vi "Measure Q.vi"(8 "error in (no error)":errorcluster, 11 "Hardware Parameters":T1={"Scan Calibration [G/V]"=0.0, "Modulation Calibration [G/V]"=0.0, "Modulation Phase [deg]"=0.0, "Modulation Frequency [Hz]"=0.0, "Attenuation [dB]"=0, "Input Channel Count"=0, "Time constant"=7, "Sensitivity"=17, "Frequency Output Voltage [V]"=0.0, "Phase Output Voltage [V]"=0.0, "Lock-in Offset Compensation"=FALSE, "RF [GHz]"=0.0, "Q Start"=0.0, "Q End"=0.0, "Balance"=0.0, "Phase Error"=0.0, "AFC Error"=0.0, "AFC"=FALSE, "Magnet Rotation"=FALSE, "Balance Scaling Factor"=1.0, "Phase Error Scaling Factor"=1.0, "AFC Error Scaling Factor"=1.0, "Frequency Counter ID"="", "Sweep Waveform"=enum."Sawtooth", "Q-Factor Scale"=0.0, " Q-Data Scale"=0.0, " Q-Data Offset"=0.0, "Magnet Rotation Slope"=0.0, "Magnet Rotation Offset"=0.0, "Phase Sweep Resolution"=0.0, "Hardware Version Number"="", "Spectrometer ID Number"=0, "Spectrometer Name"="", "Lock in Saturation"=0.0, "Balance Threshold"=0.0, "Phase Error Threshold"=0.0, "AFC Error Threshold"=0.0, "Linear Actuator Length"=0.0, "Lock-in OK?"=FALSE, "Ignore Lock-in Comm. Failure"=FALSE, "Gradient Addresses"=[], "Gradient Calibrations [G/A*mm]"=[], "Gradient Power Supplies"=[], "Lock-in Address"="", "Magnet Type"=enum."RRI", "Camera Names"=[], "Sweep Limit [Gauss]"=0.0, "Modulation Limit [Gauss]"=0.0, "Balance Threshold Exceeded?"=FALSE, "Phase Threshold Exceeded?"=FALSE, "AFC Threshold Exceeded?"=FALSE, "Consecutive Re-tune attempts"=0, "Reverse Sweep Slope [sec]"=0.0, "Reverse Sweep Offset [G]"=0.0, "AFC Field Correction [V/MHz]"=0.0, "Active Gradients (X Y Z)"=[], "SpO2 Calibration [SpO2/V]"=1.0, "Heart Rate Calibration [BPM/V]"=1.0, "Thermocouple Channel"=""} {"Sensitivity" items=["", "2 nV", "5 nV", "10 nV", "20 nV", "50 nV", "100 nV", "200 nV", "500 nV", "1 uV", "2 uV", "5 uV", "10 uV", "20 uV", "50 uV", "100 uV", "200 uV", "500 uV", "1 mV", "2 mV", "5 mV", "10 mV", "20 mV", "50 mV", "100 mV", "200 mV", "500 mV", "1 V"]; "Time constant" items=["10 us", "20 us", "40 us", "80 us", "160 us", "320 us", "640 us", "5 ms", "10 ms", "20 ms", "50 ms", "100 ms", "200 ms", "500 ms", "1 s", "2 s", "5 s", "10 s", "20 s", "50 s", "100 s", "200 s", "500 s", "1 ks", "2 ks", "5 ks", "10 ks", "20 ks", "50 ks", "100 ks"]}) -> (0 "error out":errorcluster, 2 "Q Factor":dbl, 3 "Hardware Parameters Out":T1={"Scan Calibration [G/V]"=0.0, "Modulation Calibration [G/V]"=0.0, "Modulation Phase [deg]"=0.0, "Modulation Frequency [Hz]"=0.0, "Attenuation [dB]"=0, "Input Channel Count"=0, "Time constant"=7, "Sensitivity"=17, "Frequency Output Voltage [V]"=0.0, "Phase Output Voltage [V]"=0.0, "Lock-in Offset Compensation"=FALSE, "RF [GHz]"=0.0, "Q Start"=0.0, "Q End"=0.0, "Balance"=0.0, "Phase Error"=0.0, "AFC Error"=0.0, "AFC"=FALSE, "Magnet Rotation"=FALSE, "Balance Scaling Factor"=1.0, "Phase Error Scaling Factor"=1.0, "AFC Error Scaling Factor"=1.0, "Frequency Counter ID"="", "Sweep Waveform"=enum."Sawtooth", "Q-Factor Scale"=0.0, " Q-Data Scale"=0.0, " Q-Data Offset"=0.0, "Magnet Rotation Slope"=0.0, "Magnet Rotation Offset"=0.0, "Phase Sweep Resolution"=0.0, "Hardware Version Number"="", "Spectrometer ID Number"=0, "Spectrometer Name"="", "Lock in Saturation"=0.0, "Balance Threshold"=0.0, "Phase Error Threshold"=0.0, "AFC Error Threshold"=0.0, "Linear Actuator Length"=0.0, "Lock-in OK?"=FALSE, "Ignore Lock-in Comm. Failure"=FALSE, "Gradient Addresses"=[], "Gradient Calibrations [G/A*mm]"=[], "Gradient Power Supplies"=[], "Lock-in Address"="", "Magnet Type"=enum."RRI", "Camera Names"=[], "Sweep Limit [Gauss]"=0.0, "Modulation Limit [Gauss]"=0.0, "Balance Threshold Exceeded?"=FALSE, "Phase Threshold Exceeded?"=FALSE, "AFC Threshold Exceeded?"=FALSE, "Consecutive Re-tune attempts"=0, "Reverse Sweep Slope [sec]"=0.0, "Reverse Sweep Offset [G]"=0.0, "AFC Field Correction [V/MHz]"=0.0, "Active Gradients (X Y Z)"=[], "SpO2 Calibration [SpO2/V]"=1.0, "Heart Rate Calibration [BPM/V]"=1.0, "Thermocouple Channel"=""} {"Sensitivity" items=["", "2 nV", "5 nV", "10 nV", "20 nV", "50 nV", "100 nV", "200 nV", "500 nV", "1 uV", "2 uV", "5 uV", "10 uV", "20 uV", "50 uV", "100 uV", "200 uV", "500 uV", "1 mV", "2 mV", "5 mV", "10 mV", "20 mV", "50 mV", "100 mV", "200 mV", "500 mV", "1 V"]; "Time constant" items=["10 us", "20 us", "40 us", "80 us", "160 us", "320 us", "640 us", "5 ms", "10 ms", "20 ms", "50 ms", "100 ms", "200 ms", "500 ms", "1 s", "2 s", "5 s", "10 s", "20 s", "50 s", "100 s", "200 s", "500 s", "1 ks", "2 ks", "5 ks", "10 ks", "20 ks", "50 ks", "100 ks"]})   [LabVIEW 2016]
uses:
  Types/Hardware Parameters.ctl
  <vilib>/Analysis/baseanly.llb/Mean (DBL).vi
  <vilib>/Analysis/NI_AALBase.lvlib
panel:
  out "size(s)":i32
  out "Frequency Voltage":dbl
  in  "Narrow sweep":dbl=1.0
  out "Voltage Input":dbl=9.98
  in  "Wide sweep":dbl=10.0
  out "XY Graph":cluster{"Y":dbl[], "Y":dbl[]}[](graph)
  out "Balance":dbl=-3.95030517578125
  # "Bridge I/O"
  # "Magnet Rotation"
  # "Field Calibration"
  # "Lock In Amplifier"
  # "Spectrometer Information"
  # "DAQ Settings"
  # "Gradient Coils and Field"
  # "X"
  # "Y"
  # "Z"
  # "Q-Measurements"
  # "Bridge I/O"
  # "Magnet Rotation"
  # "Field Calibration"
  # "Lock In Amplifier"
  # "Spectrometer Information"
  # "DAQ Settings"
  # "Gradient Coils and Field"
  # "X"
  # "Y"
  # "Z"
  # "Q-Measurements"
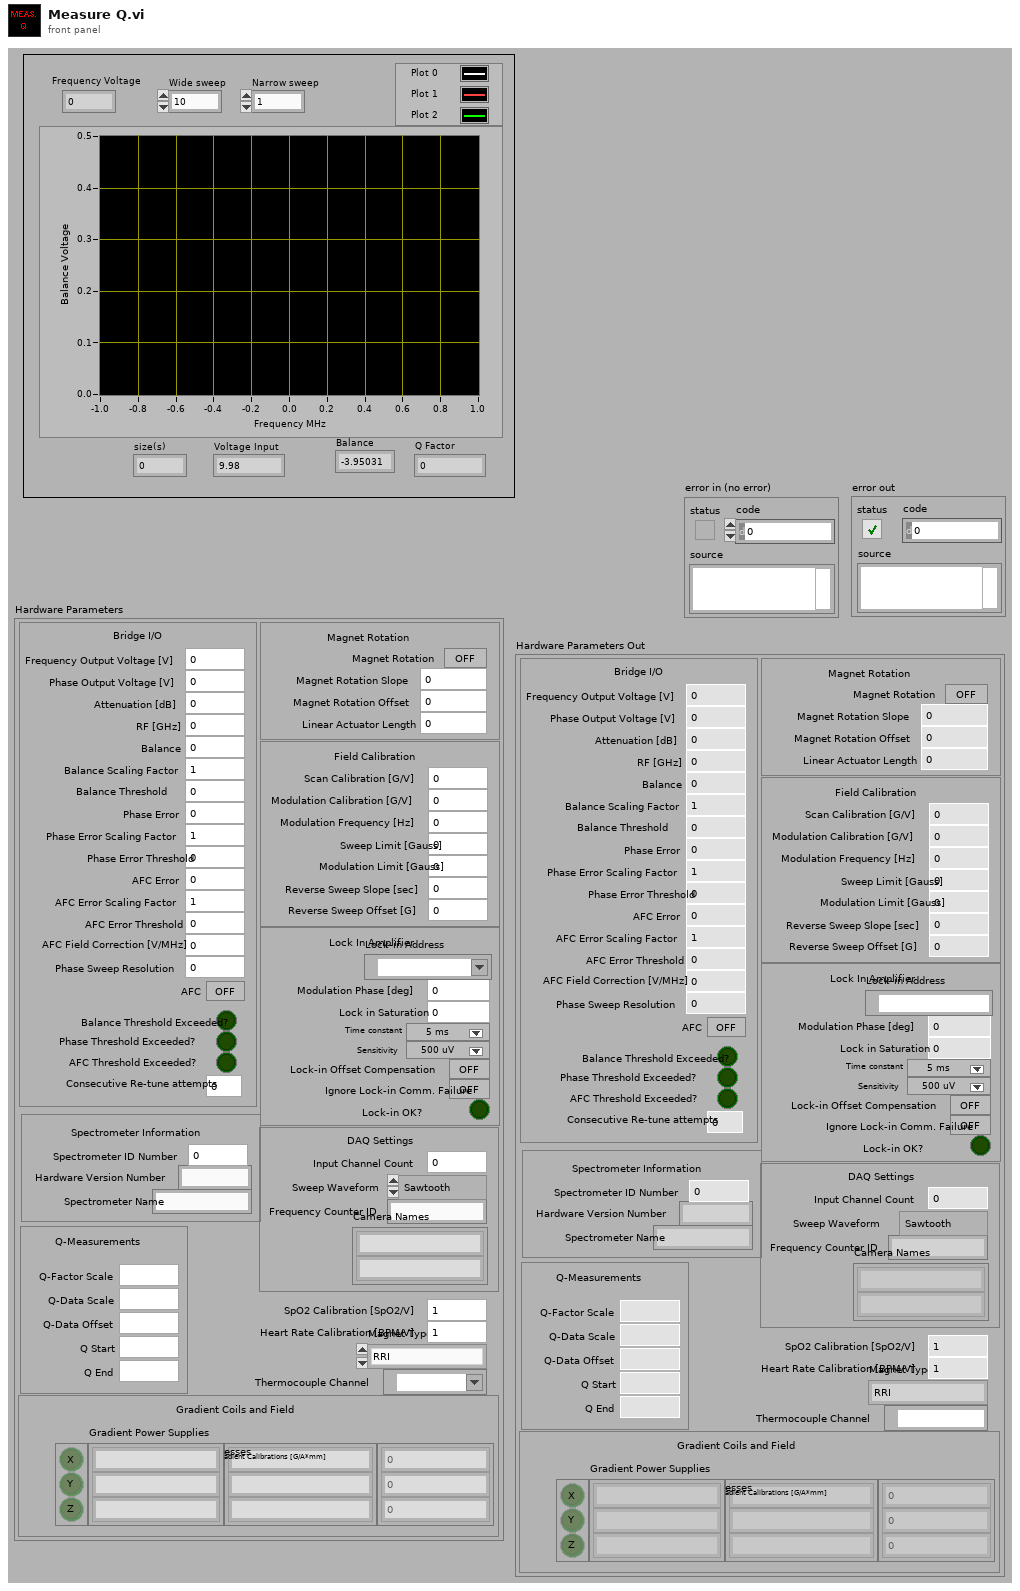
[diagram p1: front panel]
types:
  T1 = typedef "Hardware Parameters.ctl" = cluster{"Scan Calibration [G/V]":dbl, "Modulation Calibration [G/V]":dbl, "Modulation Phase [deg]":dbl, "Modulation Frequency [Hz]":dbl, "Attenuation [dB]":u16, "Input Channel Count":i32, "Time constant":u16, "Sensitivity":u16, "Frequency Output Voltage [V]":dbl, "Phase Output Voltage [V]":dbl, "Lock-in Offset Compensation":bool, "RF [GHz]":dbl, "Q Start":dbl, "Q End":dbl, "Balance":dbl, "Phase Error":dbl, "AFC Error":dbl, "AFC":bool, "Magnet Rotation":bool, "Balance Scaling Factor":dbl, "Phase Error Scaling Factor":dbl, "AFC Error Scaling Factor":dbl, "Frequency Counter ID":string, "Sweep Waveform":enum16{"Sine Wave", "Square Wave", "Sawtooth", "Triangle Wave"}, "Q-Factor Scale":dbl, " Q-Data Scale":dbl, " Q-Data Offset":dbl, "Magnet Rotation Slope":dbl, "Magnet Rotation Offset":dbl, "Phase Sweep Resolution":dbl, "Hardware Version Number":string, "Spectrometer ID Number":i32, "Spectrometer Name":string, "Lock in Saturation":dbl, "Balance Threshold":dbl, "Phase Error Threshold":dbl, "AFC Error Threshold":dbl, "Linear Actuator Length":dbl, "Lock-in OK?":bool, "Ignore Lock-in Comm. Failure":bool, "Gradient Addresses":string[], "Gradient Calibrations [G/A*mm]":dbl[], "Gradient Power Supplies":string[], "Lock-in Address":refnum<visa-resource-name>, "Magnet Type":enum16{"RRI", "BARDA", "Whole Body Permanent", "RRI Electromagnet"}, "Camera Names":string[], "Sweep Limit [Gauss]":dbl, "Modulation Limit [Gauss]":dbl, "Balance Threshold Exceeded?":bool, "Phase Threshold Exceeded?":bool, "AFC Threshold Exceeded?":bool, "Consecutive Re-tune attempts":i32, "Reverse Sweep Slope [sec]":dbl, "Reverse Sweep Offset [G]":dbl, "AFC Field Correction [V/MHz]":dbl, "Active Gradients (X Y Z)":bool[], "SpO2 Calibration [SpO2/V]":dbl, "Heart Rate Calibration [BPM/V]":dbl, "Thermocouple Channel":tag}
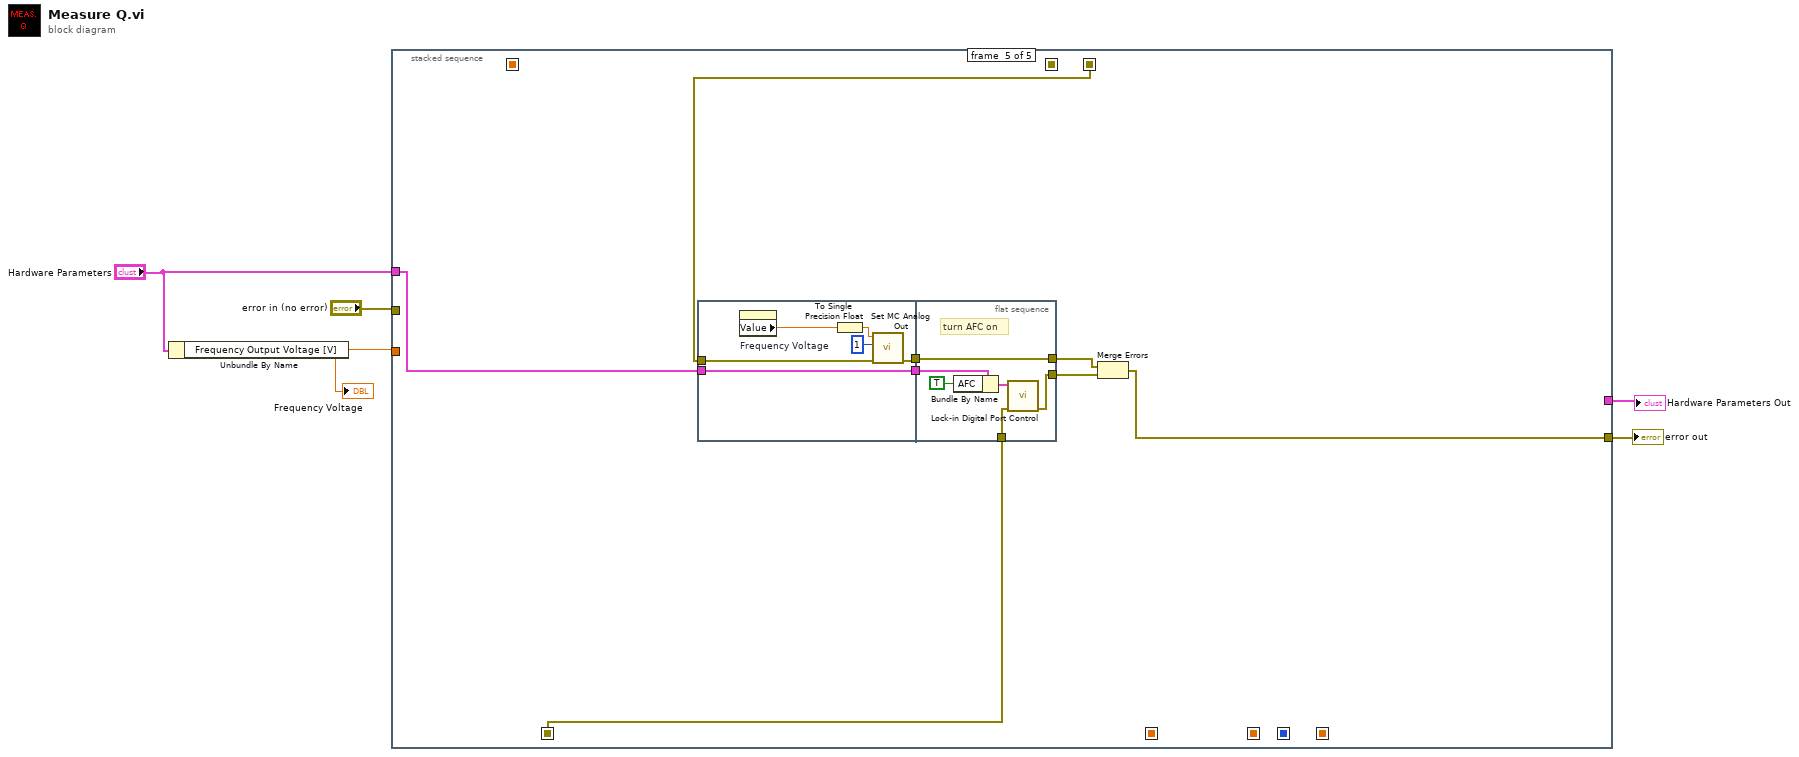
[diagram p0: block diagram]
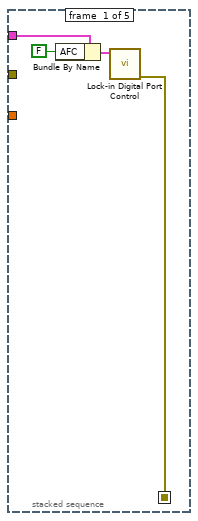
[diagram p2: hidden frame]
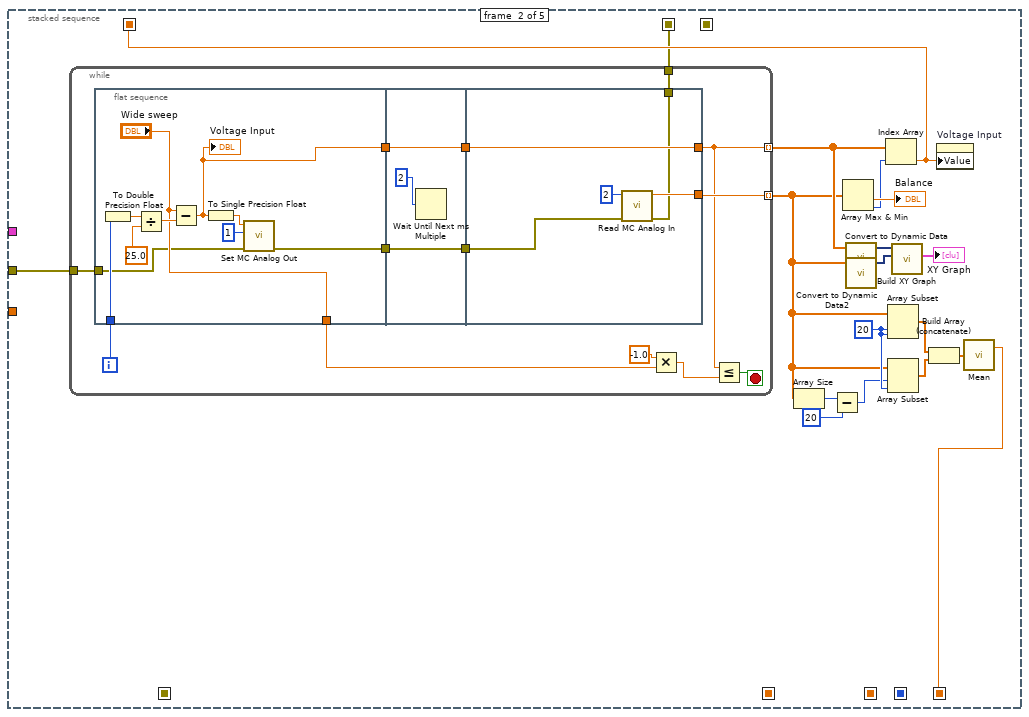
[diagram p3: hidden frame]
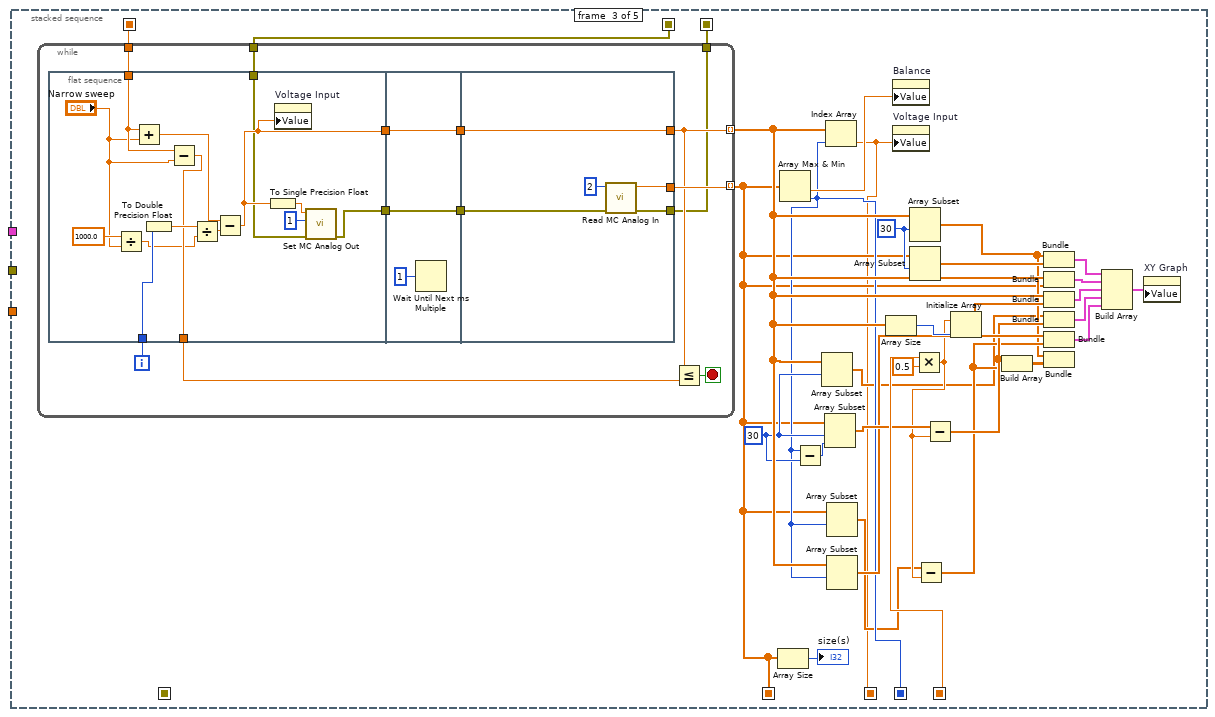
[diagram p4: hidden frame]
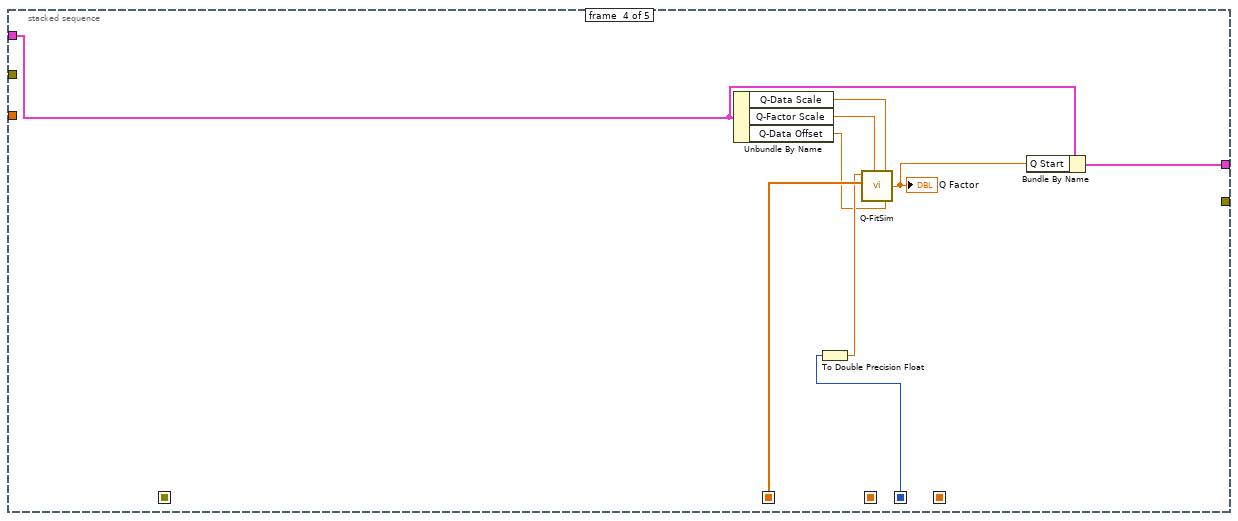
[diagram p5: hidden frame]
diagram:
  n1 = Unbundle By Name("Hardware Parameters") -> ("Frequency Output Voltage [V]"=w4:dbl)
  "Frequency Voltage" <- w4
  n2 = stacked-sequence {
    seq-local: [_ _ w61 _ _] -> [_ _ _ _ _]
    seq-local: [_ w16 _ _ _] -> [_ _ w79 _ _]
    seq-local: [_ w17 _ _ _] -> [_ _ w84 _ _]
    seq-local: [_ _ w62 _ _] -> [_ _ _ w133 _]
    seq-local: [_ _ w65 _ _] -> [_ _ _ w132 _]
    seq-local: [_ w10 _ _ _] -> [_ _ w60 _ _]
    seq-local: [_ _ w59 _ _] -> [_ _ _ _ w141]
    seq-local: [w6 _ _ _ _] -> [_ _ _ _ w138]
    tunnel: w4 -> [_ _ _ _ _]
    tunnel: "error in (no error)" -> [_ w11 _ _ _]
    tunnel: "Hardware Parameters" -> [w9 _ _ w127 w139]
    tunnel: [_ _ _ w125 _] -> w2
    tunnel: [_ _ _ _ w134] -> w1
    frame #0 {
      n3 = Bundle By Name(cluster=w9, "AFC"=FALSE) -> (w8:T1)
      n4 = call "Lock-in Digital Port Control.vi"("Hardware Parameters"=w8) -> ("error out"=w6:errorcluster)  [unwired: 10 in]
    }
    frame #1 {
      w20 = 20 ("index")
      n5 = while {
        tunnel: [w39] -> w12 mode=indexing
        tunnel: [w35] -> w18 mode=indexing
        tunnel: w11 -> [w31]
        tunnel: [w28] -> w10
        i -> [w40]
        stop <- w34 stop-if-true
        n6 = flat-sequence {
          tunnel: [w43] -> w33
          tunnel: ["Wide sweep"] -> w38
          tunnel: w40 -> [w50]
          tunnel: w31 -> [w42]
          tunnel: [w41] -> w29
          tunnel: w33 -> [w53]
          tunnel: [w53] -> w32
          tunnel: [w51] -> w30
          tunnel: w29 -> [w51]
          tunnel: [w56] -> w39
          tunnel: w32 -> [w58]
          tunnel: [w58] -> w35
          tunnel: w30 -> [w55]
          tunnel: [w54] -> w28
          frame #0 {
            n7 = To Double Precision Float(number=w50) -> (double precision float=w47:dbl)
            n8 = Divide(x=w47, y=25.0) -> (x/y=w49:dbl)
            n9 = Subtract(x="Wide sweep", y=w49) -> (x-y=w43:dbl)
            "Voltage Input" <- w43
            n10 = To Single Precision Float(number=w43) -> (single precision float=w44:sgl)
            n11 = call "Set MC Analog Out.vi"("error in (no error)"=w42, "Channel"=1, "Output Voltage"=w44) -> ("error out"=w41:errorcluster)  [unwired: 8 in]
          }
          frame #1 {
            n12 = Wait Until Next ms Multiple(millisecond multiple=u32 2 ("Inner Loop")) -> ()  [unwired: 1 out]
          }
          frame #2 {
            n13 = call "Read MC Analog In.vi"("error in (no error)"=w55, "channel"=2) -> ("error out"=w54:errorcluster, "Voltage Input"=w56:dbl)  [unwired: 8 in]
          }
        }
        n14 = Multiply(x=-1.0, y=w38) -> (x*y=w37:dbl)
        n15 = Less Or Equal?(x=w35, y=w37) -> (x <= y?=w34:bool)
      }
      n16 = Array Size(array=w12) -> (size(s)=w15:i32)
      n17 = Subtract(x=w15, y=20) -> (x-y=w13:i32)
      n18 = Array Max & Min(array=w12) -> (min value=→"Balance":dbl, min index (indices)=w23:i32)  [unwired: 2 out]
      n19 = call "Convert to Dynamic Data"("Array"=w18) -> ("Dynamic Data Type"=w25:dynamicdata)  [unwired: 3 out]
      n20 = call "Convert to Dynamic Data2"("Array"=w12) -> ("Dynamic Data Type"=w26:dynamicdata)  [unwired: 3 out]
      n21 = Index Array(array=w18, index=w23) -> (element=w17:dbl)
      n22 = Array Subset(array=w12, index=w20, length=w20) -> (w21:dbl[])
      n23 = Array Subset(array=w12, index=w13, length=w20) -> (w22:dbl[])
      n24 = call "Build XY Graph"("Y Input"=w26, "X Input"=w25) -> ("XY Graph"=→"XY Graph":cluster{"Y":dbl[], "Y":dbl[]}[])  [unwired: 3 in, 6 out]
      n25 = Build Array (concatenate)(w21, w22) -> (w19:dbl[])
      n26 = property on="Voltage Input" class="DigNum (strict)"("Value"=w17) -> ()  [unwired: 2 in, 2 out]
      n27 = call-poly <vilib>:"Mean.vi"("X"=w19) -> ("mean"=w16:dbl)  [unwired: 1 out]
    }
    frame #2 {
      w83 = 30 ("index")
      w70 = 30 ("index")
      n28 = while {
        tunnel: [w101] -> w62 mode=indexing
        tunnel: [w100] -> w71 mode=indexing
        tunnel: w84 -> [w98]
        tunnel: w60 -> [w94]
        tunnel: [w91] -> w59
        i -> [w102]
        stop <- w99 stop-if-true
        n29 = flat-sequence {
          tunnel: [w105] -> w97
          tunnel: [w112] -> w95
          tunnel: w102 -> [w116]
          tunnel: w98 -> [w109]
          tunnel: w94 -> [w104]
          tunnel: [w103] -> w92
          tunnel: w97 -> [w119]
          tunnel: [w119] -> w96
          tunnel: [w117] -> w93
          tunnel: w92 -> [w117]
          tunnel: [w122] -> w101
          tunnel: w96 -> [w124]
          tunnel: [w124] -> w100
          tunnel: w93 -> [w121]
          tunnel: [w120] -> w91
          frame #0 {
            n30 = Divide(x=1000.0, y="Narrow sweep") -> (x/y=w110:dbl)
            n31 = Add(x=w109, y="Narrow sweep") -> (x+y=w113:dbl)
            n32 = To Double Precision Float(number=w116) -> (double precision float=w114:dbl)
            n33 = Subtract(x=w109, y="Narrow sweep") -> (x-y=w112:dbl)
            n34 = Divide(x=w114, y=w110) -> (x/y=w115:dbl)
            n35 = Subtract(x=w113, y=w115) -> (x-y=w105:dbl)
            n36 = To Single Precision Float(number=w105) -> (single precision float=w107:sgl)
            n37 = property on="Voltage Input" class="DigNum (strict)"("Value"=w105) -> ()  [unwired: 2 in, 2 out]
            n38 = call "Set MC Analog Out.vi"("error in (no error)"=w104, "Channel"=1, "Output Voltage"=w107) -> ("error out"=w103:errorcluster)  [unwired: 8 in]
          }
          frame #1 {
            n39 = Wait Until Next ms Multiple(millisecond multiple=u32 1) -> ()  [unwired: 1 out]
          }
          frame #2 {
            n40 = call "Read MC Analog In.vi"("error in (no error)"=w121, "channel"=2) -> ("error out"=w120:errorcluster, "Voltage Input"=w122:dbl)  [unwired: 8 in]
          }
        }
        n41 = Less Or Equal?(x=w100, y=w95) -> (x <= y?=w99:bool)
      }
      n42 = Array Size(array=w62) -> (size(s)=→"size(s)":i32)
      n43 = Array Max & Min(array=w62) -> (min value=w89:dbl, min index (indices)=w65:i32)  [unwired: 2 out]
      n44 = Subtract(x=w65, y=w70) -> (x-y=w76:i32)
      n45 = Array Subset(array=w71, index=w70) -> (w64:dbl[])  [unwired: 1 in]
      n46 = Array Subset(array=w62, index=w70, length=w76) -> (w77:dbl[])
      n47 = Index Array(array=w71, index=w65) -> (element=w61:dbl)
      n48 = Array Subset(array=w62, index=w65) -> (w63:dbl[])  [unwired: 1 in]
      n49 = Array Subset(array=w71, index=w65) -> (w74:dbl[])  [unwired: 1 in]
      n50 = Array Size(array=w71) -> (size(s)=w86:i32)
      n51 = property on="Balance" class="DigNum (strict)"("Value"=w89) -> ()  [unwired: 2 in, 2 out]
      n52 = property on="Voltage Input" class="DigNum (strict)"("Value"=w61) -> ()  [unwired: 2 in, 2 out]
      n53 = Array Subset(array=w71, index=w83) -> (w66:dbl[])  [unwired: 1 in]
      n54 = Array Subset(array=w62, index=w83) -> (w82:dbl[])  [unwired: 1 in]
      n55 = Multiply(x=w79, y=0.5) -> (x*y=w73:dbl)
      n56 = Subtract(x=w63, y=w73) -> (x-y=w68:dbl[])
      n57 = Subtract(x=w77, y=w73) -> (x-y=w69:dbl[])
      n58 = Initialize Array(w73, w86) -> (w85:dbl[])
      n59 = Build Array(w69, w68) -> (w67:dbl[][])
      n60 = Bundle(w66, w82) -> (w81:cluster{dbl[], dbl[]})  [unwired: 1 in]
      n61 = Bundle(w71, w62) -> (w80:cluster{dbl[], dbl[]})  [unwired: 1 in]
      n62 = Bundle(w71, w85) -> (w87:cluster{dbl[], dbl[]})  [unwired: 1 in]
      n63 = Bundle(w64, w69) -> (w78:cluster{dbl[], dbl[]})  [unwired: 1 in]
      n64 = Bundle(w74, w68) -> (w75:cluster{dbl[], dbl[]})  [unwired: 1 in]
      n65 = Bundle(w66, w67) -> ()  [unwired: 1 in, 1 out]
      n66 = Build Array(w81, w80, w87, w78, w75) -> (w88:cluster{dbl[], dbl[]}[])
      n67 = property on="XY Graph" class="XYGraph (strict)"("Value"=w88) -> ()  [unwired: 2 in, 2 out]
    }
    frame #3 {
      n68 = Unbundle By Name(w127) -> ("Q-Data Scale"=w130:dbl, "Q-Factor Scale"=w129:dbl, "Q-Data Offset"=w128:dbl)
      n69 = To Double Precision Float(number=w132) -> (double precision float=w131:dbl)
      n70 = call "Q-FitSim.vi"("Center Frequency"=w131, "Raw Data"=w133, "Q-Scale"=w129, "Q -Data Scale"=w130, "Q-Data Offset"=w128) -> ("Q"=w126:dbl)  [unwired: 2 in]
      "Q Factor" <- w126
      n71 = Bundle By Name(cluster=w127, "Q Start"=w126) -> (w125:T1)
    }
    frame #4 {
      n72 = flat-sequence {
        tunnel: w141 -> [w144]
        tunnel: [w143] -> w140
        tunnel: w139 -> [w143]
        tunnel: [w142] -> w137
        tunnel: w140 -> [w151]
        tunnel: w138 -> [w150]
        tunnel: w137 -> [w149]
        tunnel: [w149] -> w136
        tunnel: [w148] -> w135
        frame #0 {
          n73 = property on="Frequency Voltage" class="DigNum (strict)"() -> ("Value"=w145:dbl)  [unwired: 2 in, 2 out]
          n74 = To Single Precision Float(number=w145) -> (single precision float=w146:sgl)
          n75 = call "Set MC Analog Out.vi"("error in (no error)"=w144, "Channel"=1, "Output Voltage"=w146) -> ("error out"=w142:errorcluster)  [unwired: 8 in]
        }
        frame #1 {
          # "turn AFC on"
          n76 = Bundle By Name(cluster=w151, "AFC"=TRUE) -> (w153:T1)
          n77 = call "Lock-in Digital Port Control.vi"("error in (no error)"=w150, "Hardware Parameters"=w153) -> ("error out"=w148:errorcluster)  [unwired: 9 in]
        }
      }
      n78 = Merge Errors(w136, w135) -> (w134:errorcluster)
    }
  }
  "Hardware Parameters Out" <- w2
  "error out" <- w1
